vi "Status.Builder.Set State.vi"(10 "Builder State":refnum<class "Status.Builder.State.lvclass">, 11 "Status.Builder in":refnum<class "Status.Builder.lvclass">) -> (3 "Status.Builder out":refnum<class "Status.Builder.lvclass">)   [LabVIEW 2016, in "DSF.Engine.lvlib" / "Status.Builder.lvclass"]
uses:
  Status.Builder.lvclass
  Status.Builder.State.lvclass
  Status.Builder.lvclass/Status.Builder.ctl
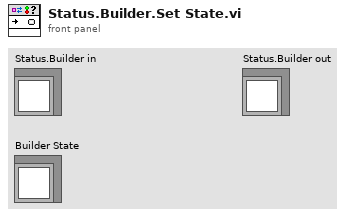
[diagram p1: front panel]
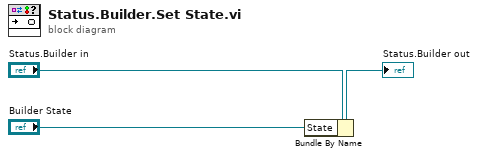
[diagram p0: block diagram]
diagram:
  n1 = Bundle By Name(cluster="Status.Builder in", "State"="Builder State") -> (→"Status.Builder out":refnum<class "Status.Builder.lvclass">)
